vi "Steering Power PID (SubVI).vi"(5 "rightFrontAngleError":dbl, 9 "leftFrontAngleError":dbl, 11 "moduleAbsoluteAngles":T1, 12 "leftRearAngleError":dbl, 14 "rightRearAngleError":dbl) -> (3 "overriden":bool, 4 "rightFrontSteeringPower":dbl, 6 "leftFrontSteeringPower":dbl, 10 "leftRearSteeringPower":dbl, 15 "rightRearSteeringPower":dbl)   [LabVIEW 2020]
uses:
  TypeDefs/Absolute Angle TypeDef.ctl
  <vilib>/addons/control/pid/pid.llb/PID (DBL).vi
  <vilib>/addons/control/pid/NI_PID_pid.lvlib
panel:
  out "rightFrontAngleError":dbl(graph)
  out "rightFrontoutput":dbl(graph)
  out "rightRearAngle":dbl(graph)
  out "rightFrontAngle":dbl(graph)
  out "leftRearAngle":dbl(graph)
  out "leftFrontAngle":dbl(graph)
  in  "Setpoint":dbl
  in  "Overrie - PID Tune":bool
  in  "FeedFoward":dbl
  in  "Kp":dbl=0.01
  in  "Kd":dbl=0.001
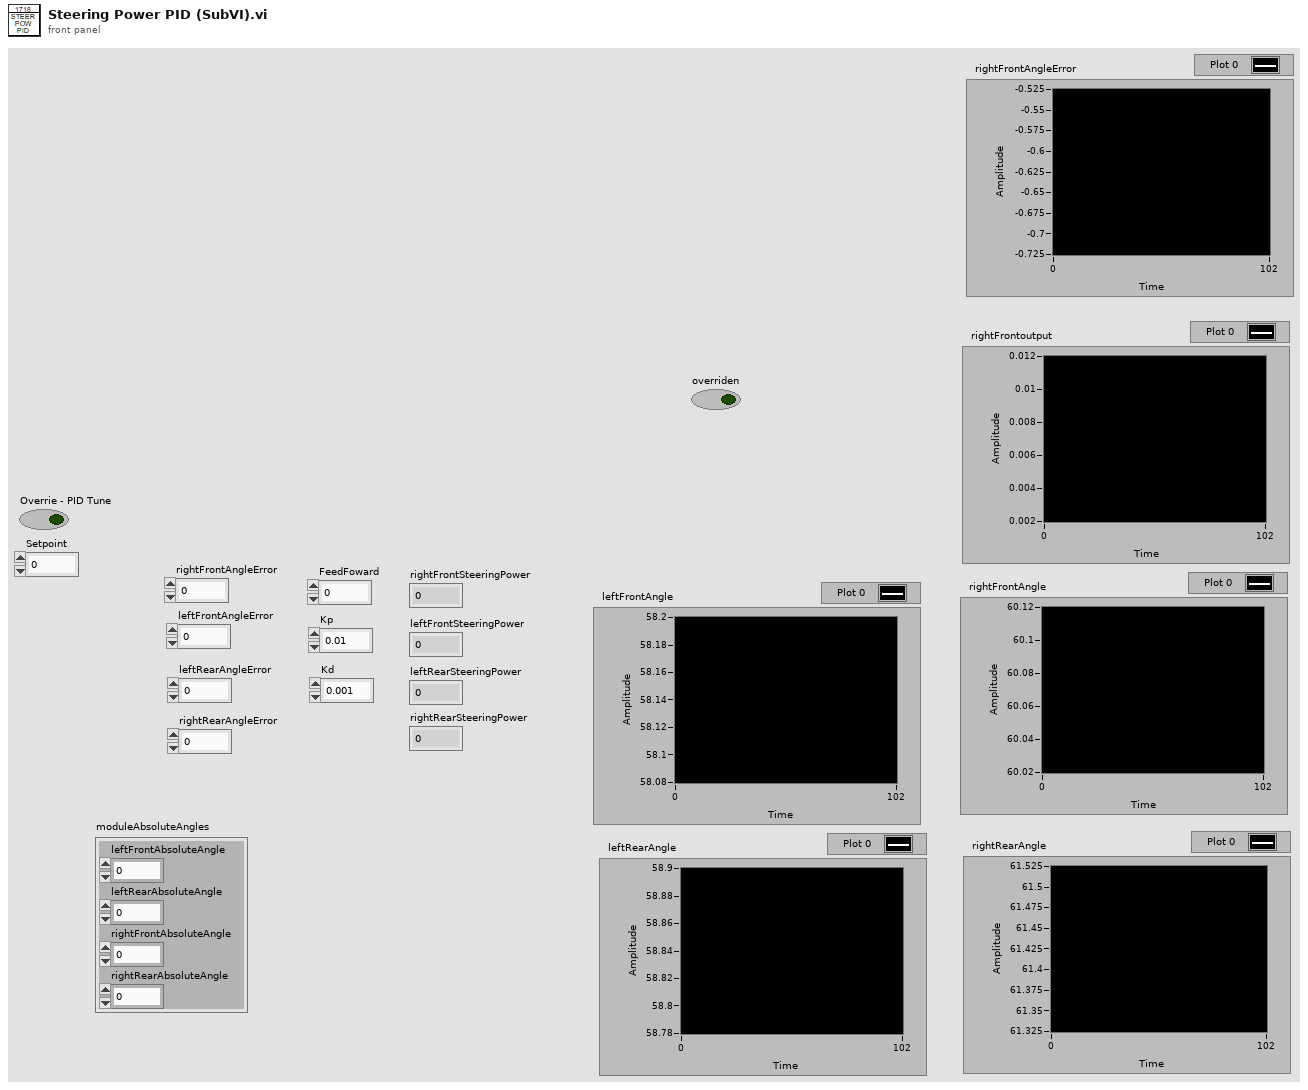
[diagram p1: front panel]
types:
  T1 = typedef "Absolute Angle TypeDef.ctl" = cluster{"leftFrontAbsoluteAngle":dbl, "leftRearAbsoluteAngle":dbl, "rightFrontAbsoluteAngle":dbl, "rightRearAbsoluteAngle":dbl}
  T2 = cluster{"proportional gain (Kc)":dbl, "integral time (Ti, min)":dbl, "derivative time (Td, min)":dbl}
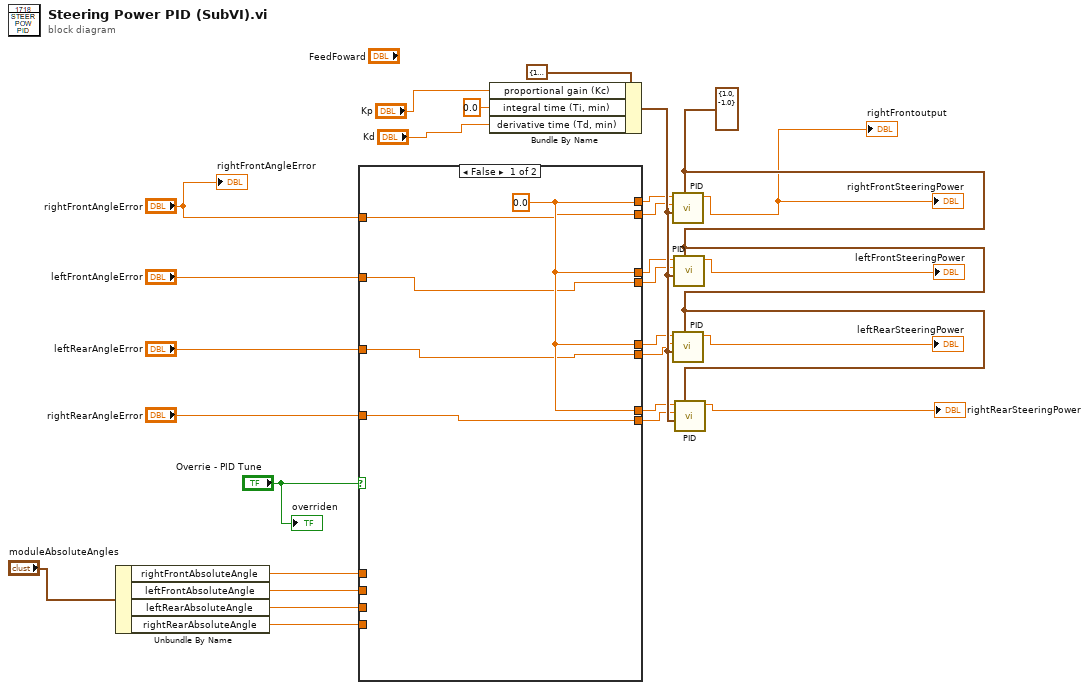
[diagram p0: block diagram]
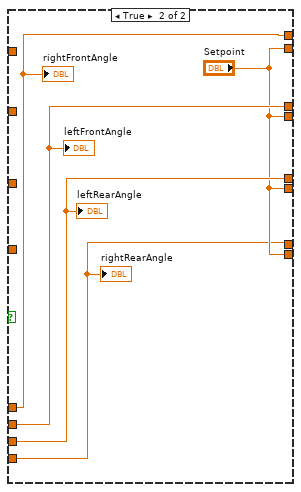
[diagram p2: hidden frame]
diagram:
  w3 = cluster{"output high":dbl, "output low":dbl} {"output high"=1.0, "output low"=-1.0} ("output range")
  n1 = Unbundle By Name("moduleAbsoluteAngles") -> ("rightFrontAbsoluteAngle"=w26:dbl, "leftFrontAbsoluteAngle"=w25:dbl, "leftRearAbsoluteAngle"=w24:dbl, "rightRearAbsoluteAngle"=w23:dbl)
  n2 = case shown="False" "Overrie - PID Tune" {
    tunnel: [w33 w38] -> w11
    tunnel: [w33 w37] -> w9
    tunnel: [w33 w36] -> w7
    tunnel: [w33 w34] -> w5
    tunnel: [w32 "Setpoint"] -> w10
    tunnel: w26 -> [_ w38]
    tunnel: [w31 "Setpoint"] -> w8
    tunnel: w25 -> [_ w37]
    tunnel: [w30 "Setpoint"] -> w6
    tunnel: w24 -> [_ w36]
    tunnel: [w29 "Setpoint"] -> w4
    tunnel: w23 -> [_ w34]
    tunnel: "rightFrontAngleError" -> [w32 _]
    tunnel: "leftFrontAngleError" -> [w31 _]
    tunnel: "leftRearAngleError" -> [w30 _]
    tunnel: "rightRearAngleError" -> [w29 _]
    frame False {
      w33 = 0.0 ("Setpoint")
    }
    frame True {
      "leftFrontAngle" <- w37
      "rightFrontAngle" <- w38
      "leftRearAngle" <- w36
      "rightRearAngle" <- w34
    }
  }
  n3 = Bundle By Name(cluster=T2 {"proportional gain (Kc)"=1.0, "integral time (Ti, min)"=0.01, "derivative time (Td, min)"=0.0} ("PID gains"), "proportional gain (Kc)"="Kp", "integral time (Ti, min)"=0.0, "derivative time (Td, min)"="Kd") -> (w12:T2)
  n4 = call-poly <vilib>:"PID.vi"("output range"=w3, "PID gains"=w12, "process variable"=w10, "setpoint"=w11) -> ("output"=→"rightFrontSteeringPower" →"rightFrontoutput":dbl)  [unwired: 6 in, 1 out]
  n5 = call-poly <vilib>:"PID.vi"("output range"=w3, "PID gains"=w12, "process variable"=w6, "setpoint"=w7) -> ("output"=→"leftRearSteeringPower":dbl)  [unwired: 6 in, 1 out]
  n6 = call-poly <vilib>:"PID.vi"("output range"=w3, "PID gains"=w12, "process variable"=w8, "setpoint"=w9) -> ("output"=→"leftFrontSteeringPower":dbl)  [unwired: 6 in, 1 out]
  n7 = call-poly <vilib>:"PID.vi"("output range"=w3, "PID gains"=w12, "process variable"=w4, "setpoint"=w5) -> ("output"=→"rightRearSteeringPower":dbl)  [unwired: 6 in, 1 out]
  "overriden" <- "Overrie - PID Tune"
  "rightFrontAngleError" <- "rightFrontAngleError"
